vi "A Encoder to distance.vi"(0 "Middle Left Encoder Value":dbl, 1 "Middle Right Encoder Value":dbl, 3 "Desired Distance (in)":dbl) -> (8 "Got to position?":bool)   [LabVIEW 2015]
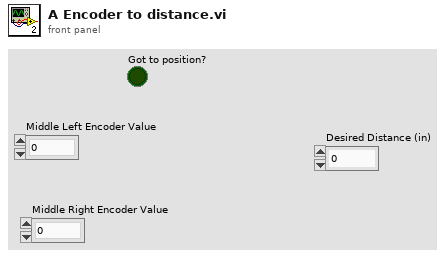
[diagram p1: front panel]
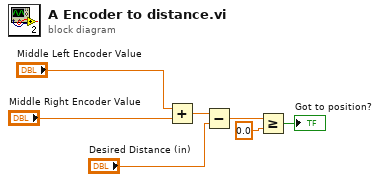
[diagram p0: block diagram]
diagram:
  n1 = Add(x="Middle Left Encoder Value", y="Middle Right Encoder Value") -> (x+y=w2:dbl)
  n2 = Subtract(x=w2, y="Desired Distance (in)") -> (x-y=w3:dbl)
  n3 = Greater Or Equal?(x=w3, y=0.0) -> (x >= y?=→"Got to position?":bool)
